vi "Config Zero Point.vi"(0 "VISA resource name":refnum<visa-resource-name>, 5 "Capacitance (0 pF)":dbl min=-99999999.0 max=99999999.0 format="%#_10f", 7 "Loss (0 jpF)":dbl min=-99999999.0 max=99999999.0 format="%#_10f", 9 "Frequency (1000 Hz)":dbl=1000.0 min=-99999999.0 max=99999999.0 format="%#_10f", 11 "error in":errorcluster) -> (4 "VISA resource name out":refnum<visa-resource-name>, 15 "error out":errorcluster)   [LabVIEW 2019, in "Andeen-Hagerling 2700(400 firmware).lvlib"]
doc: "Provides a manual way to enter capacitance, loss and frequency zero compensation values."
uses:
  Andeen-Hagerling 2700(400 firmware).lvlib
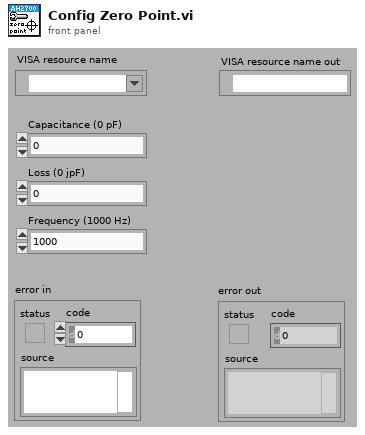
[diagram p1: front panel]
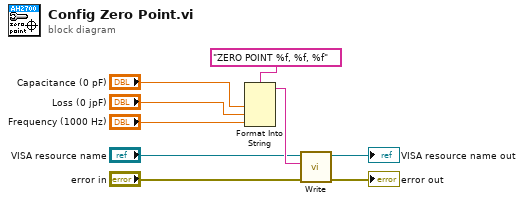
[diagram p0: block diagram]
diagram:
  n1 = Format Into String(format string="ZERO POINT %f, %f, %f", "Capacitance (0 pF)", "Loss (0 jpF)", "Frequency (1000 Hz)") -> (resulting string=w9:string)  [unwired: 2 in, 1 out]
  n2 = call "Write.vi"("error in"="error in", "command"=w9, "VISA resource name"="VISA resource name") -> ("error out"=→"error out":errorcluster, "VISA resource name out"=→"VISA resource name out":refnum<visa-resource-name>)  [unwired: 7 in]
